vi "Tarea 5.vi"() -> ()   [LabVIEW 2019]
uses:
  Student Material/Student Material/Module 2/Exercise 5/CLD 5 Data Cluster.ctl
panel:
  in  "Array In":T1[][](array[typedef])=[[{"Numeric"=2.25, "Boolean"=FALSE, "String"="One"}, {"Numeric"=1.35, "Boolean"=TRUE, "String"="Two"}, {"Numeric"=1.5, "Boolean"=FALSE, "String"="Three"}, {"Numeric"=1.0, "Boolean"=TRUE, "String"="Four"}], [{"Numeric"=2.0, "Boolean"=TRUE, "String"="Five"}, {"Numeric"=0.75, "Boolean"=FALSE, "String"="Six"}, {"Numeric"=0.9, "Boolean"=TRUE, "String"="Seven"}, {"Numeric"=0.75, "Boolean"=FALSE, "String"="Eight"}]]
  out "Array Out":T1[][](array[typedef])
  in  "Get/Set":enum16{"Get", "Set"}(ring)
  in  "error in (no error)":errorcluster
  out "error out":errorcluster
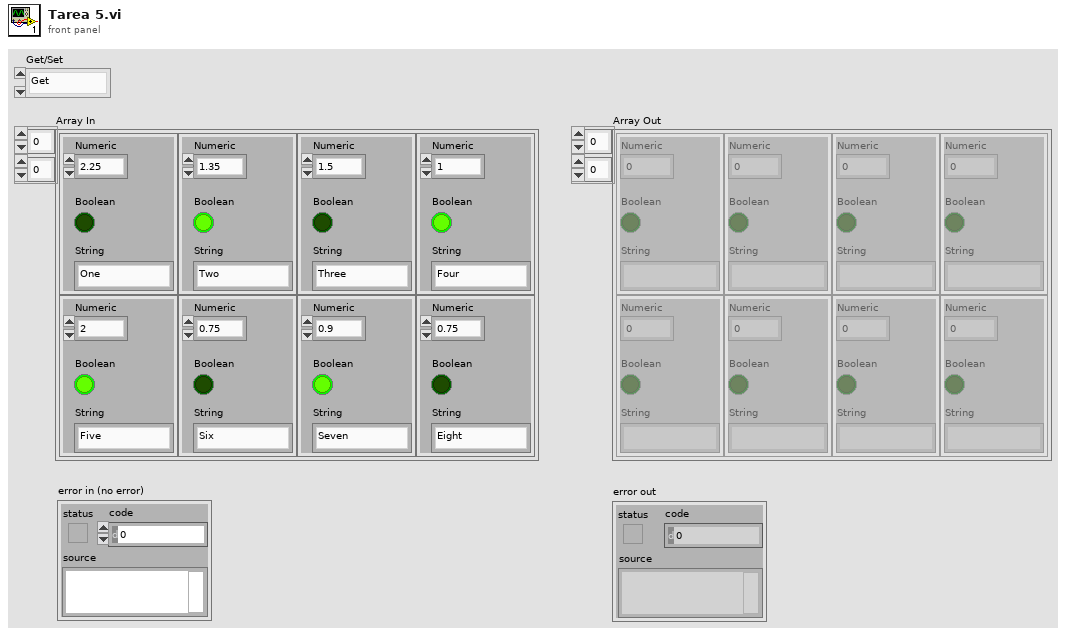
[diagram p1: front panel]
types:
  T1 = typedef "CLD 5 Data Cluster.ctl" = cluster{"Numeric":dbl, "Boolean":bool, "String":string}
  T2 = enum16{"open", "replace", "create", "open or create", "replace or create", "replace or create with confirmation"}
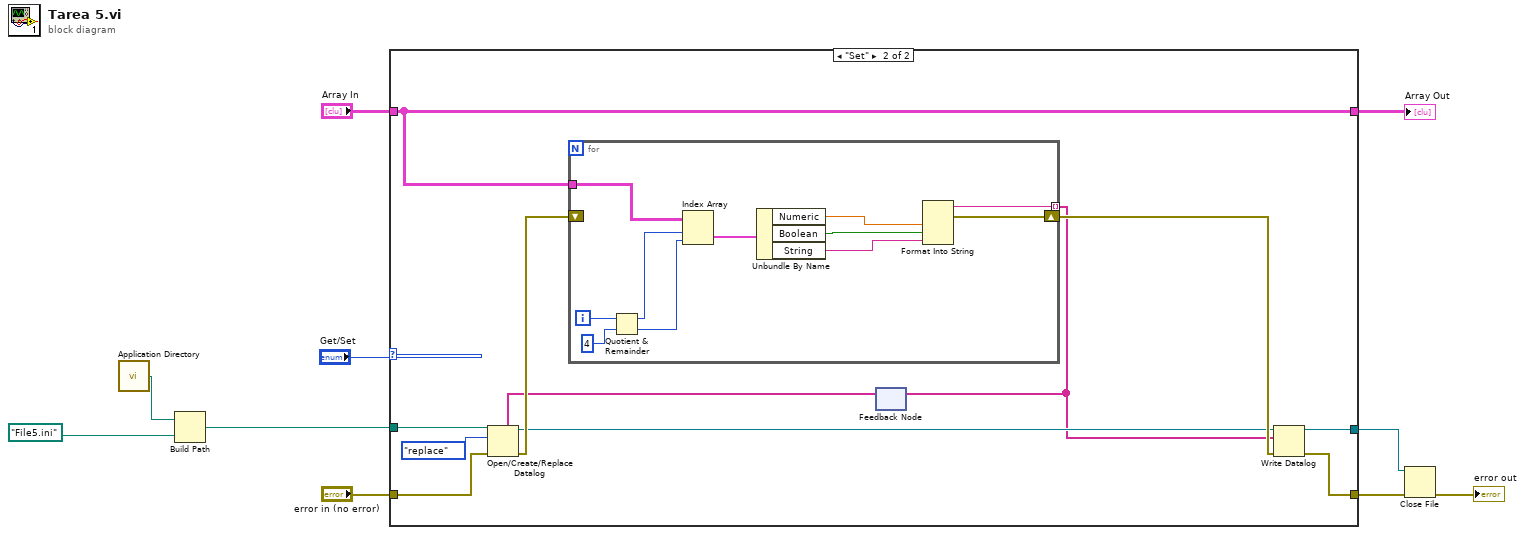
[diagram p0: block diagram]
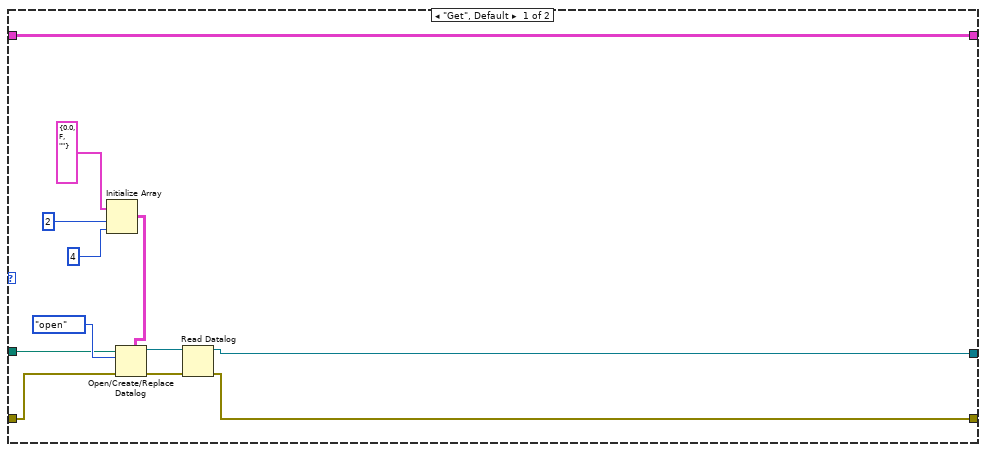
[diagram p2: hidden frame]
diagram:
  n1 = call <vilib>:"Application Directory.vi"() -> ("Application Directory"=w4:path)
  n2 = Build Path(base path=w4, name or relative path=path "File5.ini") -> (appended path=w2:path)
  n3 = case shown="\"Set\"" "Get/Set" {
    tunnel: [w11 w30] -> w6
    tunnel: "error in (no error)" -> [w19 w31]
    tunnel: "Array In" -> [w22 w29]
    tunnel: w2 -> [w20 w32]
    tunnel: [w22 w29] -> w3
    tunnel: [w12 w23] -> w1
    frame "Get", Default {
      n4 = Initialize Array(T1 {"Numeric"=0.0, "Boolean"=FALSE, "String"=""} ("Array"), 2 ("dimension size"), 4 ("dimension size")) -> (w15:T1[][])
      n5 = Open/Create/Replace Datalog(5:w15, 8:w19, 10:T2."open" ("operation (0:open)"), 11:w20) -> (0:w13:errorcluster, 3:w14:refnum<k1>)  [unwired: 3 out]
      n6 = Read Datalog(4:w13, 7:w14) -> (0:w11:errorcluster, 3:w12:refnum<k1>)  [unwired: 2 out]
    }
    frame "Set" {
      n7 = feedback #1() -> (w26:string[])  [unwired: 1 in]
      n8 = Open/Create/Replace Datalog(5:w26, 8:w31, 10:T2."replace" ("operation (0:open)"), 11:w32) -> (0:w27:errorcluster, 3:w25:refnum<k1>)  [unwired: 3 out]
      n9 = for {
        tunnel: w29 -> [w44]
        shift-right: [w35] -> w28
        shift-left: w27 -> [_]
        tunnel: [w34] -> w24 mode=indexing
        i -> [w43]
        n10 = Quotient & Remainder(x=w43, y=4) -> (x-y*floor(x/y)=w41:i32, floor(x/y)=w40:i32)
        n11 = Index Array(array=w44, index (row)=w41, index (col)=w40) -> (element=w39:T1)
        n12 = Unbundle By Name(w39) -> ("Numeric"=w38:dbl, "Boolean"=w37:bool, "String"=w36:string)
        n13 = Format Into String(w38, w37, w36) -> (resulting string=w34:string, error out=w35:errorcluster)  [unwired: 3 in]
      }
      n14 = feedback-in #1(w24) -> ()
      n15 = Write Datalog(4:w28, 6:w24, 7:w25) -> (0:w30:errorcluster, 3:w23:refnum<k1>)
    }
  }
  "Array Out" <- w3
  n16 = Close File(refnum=w1, error in=w6) -> (error out=→"error out":errorcluster)  [unwired: 1 out]
